vi "Build PN (SubVI).vi"(11 "read buffer":string) -> (3 "String":string)   [LabVIEW 2017]
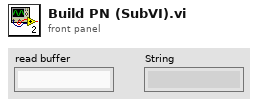
[diagram p1: front panel]
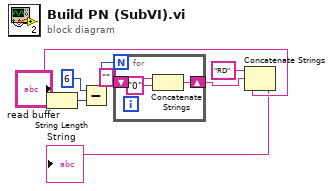
[diagram p0: block diagram]
diagram:
  n1 = String Length(string="read buffer") -> (length=w2:i32)
  n2 = Subtract(x=6, y=w2) -> (x-y=w3:i32)
  n3 = for {
    N: w3 -> [_]
    shift-right: [w11] -> w6
    shift-left: "" -> [w10]
    n4 = Concatenate Strings(w10, "0" ("string")) -> (w11:string)
  }
  n5 = Concatenate Strings("RD" ("string"), w6, "read buffer") -> (→"String":string)
